vi "oscilloscope.vi"() -> ()   [LabVIEW 2011]
panel:
  in  "filename":path
  out "Waveform Chart":dbl(graph)
  in  "InitialValue":dbl
  in  "Stop":bool
  out "FrequencyOut":dbl
  in  "Frequency":i16=2
  # "MY PROGRAM"
  # "make current\nvalue default"
  # "Exercise: Make your own program that writes floats. Each float to its own line.\nHint: Scan Value, concatenate strings"
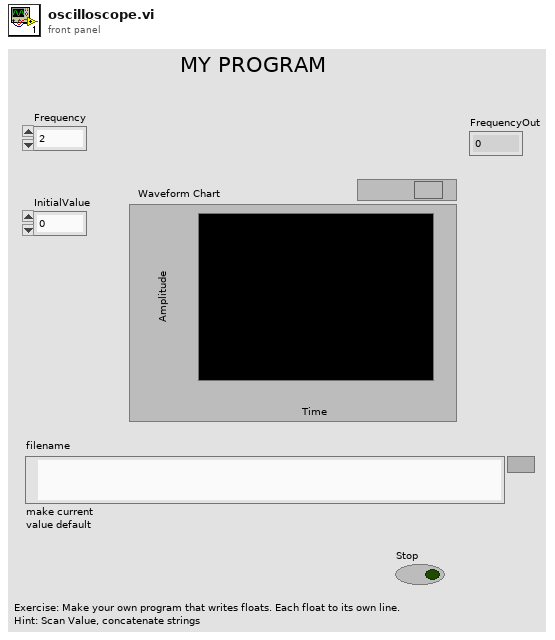
[diagram p1: front panel]
types:
  T1 = enum16{"open", "replace", "create", "open or create", "replace or create", "replace or create with confirmation"}
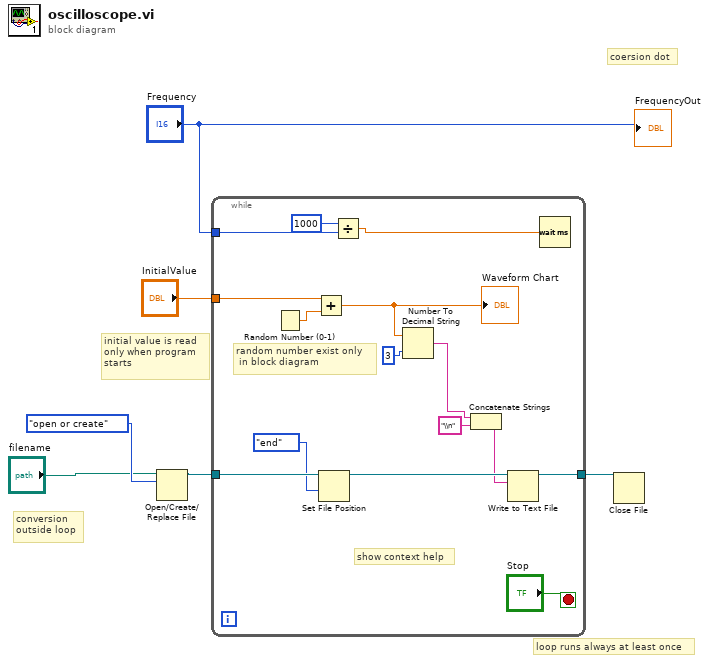
[diagram p0: block diagram]
diagram:
  # "conversion\noutside loop"
  # "initial value is read\nonly when program\nstarts"
  # "loop runs always at least once"
  # "coersion dot"
  n1 = Open/Create/Replace File(file path (use dialog)="filename", operation (0:open)=T1."open or create") -> (refnum out=w4:refnum<file>)  [unwired: 4 in, 2 out]
  n2 = while {
    tunnel: "Frequency" -> [w21]
    tunnel: "InitialValue" -> [w17]
    tunnel: w4 -> [w13]
    tunnel: [w10] -> w3
    stop <- "Stop" stop-if-true
    # "show context help"
    # "random number exist only\n in block diagram"
    n3 = Random Number (0-1)() -> (number: 0 to 1=w16:dbl)
    n4 = Add(x=w17, y=w16) -> (x+y=w15:dbl)
    "Waveform Chart" <- w15
    n5 = Set File Position(refnum=w13, from (0:start)=enum16{"start", "end", "current"}."end") -> (refnum out=w12:refnum<file>)  [unwired: 2 in, 1 out]
    n6 = Divide(x=i16 1000, y=w21) -> (x/y=w19:dbl)
    n7 = Number To Decimal String(number=w15, width (-)=i16 3) -> (decimal integer string=w9:string)
    n8 = Concatenate Strings(w9, "\\n" ("string")) -> (w8:string)
    n9 = Write to Text File(file (use dialog)=w12, text=w8) -> (refnum out=w10:refnum<file>)  [unwired: 2 in, 2 out]
    n10 = Wait (ms)(milliseconds to wait=w19) -> ()  [unwired: 1 out]
  }
  n11 = Close File(refnum=w3) -> ()  [unwired: 1 in, 2 out]
  "FrequencyOut" <- "Frequency"
